vi "Data Chart for Flow Meter Test Time Chart.vi"(0 "Initialize":bool, 5 "Data Array":dbl[](array[numeric])) -> (6 "XY Graph":T1(graph))   [LabVIEW 2009]
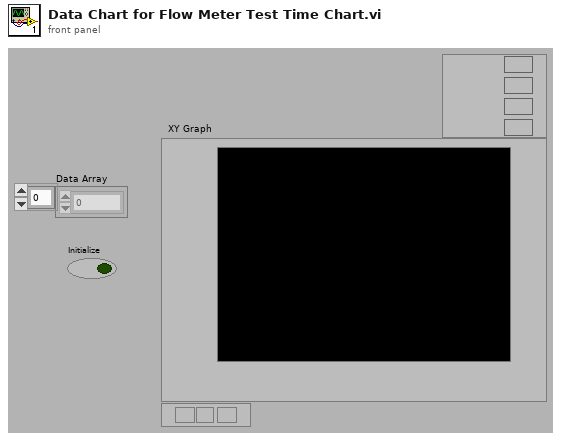
[diagram p1: front panel]
types:
  T1 = cluster{"XY chart data":cluster{"x":dbl, "y":dbl}[]}[]
  T2 = cluster{cluster{"Elapsed Time (sec)":dbl, dbl}[]}[]
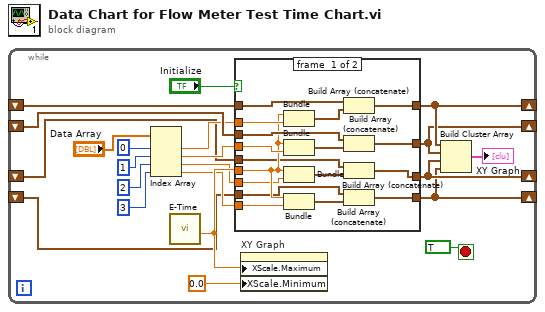
[diagram p0: block diagram]
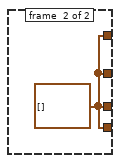
[diagram p2: hidden frame]
diagram:
  n1 = while {
    shift-right: [w21] -> _
    shift-left: _ -> [w19]
    shift-right: [w20] -> _
    shift-left: _ -> [w18]
    shift-right: [w3] -> _
    shift-left: _ -> [w5]
    shift-right: [w2] -> _
    shift-left: _ -> [w4]
    stop <- TRUE ("stop") stop-if-true
    n2 = Index Array(array="Data Array", index #1=0 ("index"), index #2=1 ("index"), index #3=2 ("index"), index #4=3 ("index")) -> (element #1=w10:dbl, element #2=w9:dbl, element #3=w7:dbl, element #4=w6:dbl)
    n3 = call "E-Time.vi"() -> ("Elapsed Time (sec)"=w8:dbl)  [unwired: 9 in, 2 out]
    n4 = case shown="False" "Initialize" {
      tunnel: [w37 w40] -> w21
      tunnel: [w36 w40] -> w20
      tunnel: w19 -> [w35 _]
      tunnel: w18 -> [w34 _]
      tunnel: w10 -> [w33 _]
      tunnel: w9 -> [w32 _]
      tunnel: w8 -> [w31 _]
      tunnel: w7 -> [w30 _]
      tunnel: w6 -> [w29 _]
      tunnel: w5 -> [w28 _]
      tunnel: w4 -> [w25 _]
      tunnel: [w24 w40] -> w3
      tunnel: [w23 w40] -> w2
      frame #0 {
        n5 = Bundle("Elapsed Time (sec)"=w31, w33) -> (w39:cluster{"Elapsed Time (sec)":dbl, dbl})  [unwired: 1 in]
        n6 = Bundle("Elapsed Time (sec)"=w31, w32) -> (w38:cluster{"Elapsed Time (sec)":dbl, dbl})  [unwired: 1 in]
        n7 = Bundle("Elapsed Time (sec)"=w31, w30) -> (w27:cluster{"Elapsed Time (sec)":dbl, dbl})  [unwired: 1 in]
        n8 = Bundle("Elapsed Time (sec)"=w31, w29) -> (w26:cluster{"Elapsed Time (sec)":dbl, dbl})  [unwired: 1 in]
        n9 = Build Array (concatenate)(w35, w39) -> (w37:cluster{"Elapsed Time (sec)":dbl, dbl}[])
        n10 = Build Array (concatenate)(w34, w38) -> (w36:cluster{"Elapsed Time (sec)":dbl, dbl}[])
        n11 = Build Array (concatenate)(w28, w27) -> (w24:cluster{"Elapsed Time (sec)":dbl, dbl}[])
        n12 = Build Array (concatenate)(w25, w26) -> (w23:cluster{"Elapsed Time (sec)":dbl, dbl}[])
      }
      frame #1 {
        w40 = cluster{"Elapsed Time (sec)":dbl, dbl}[] []
      }
    }
    n13 = property on="XY Graph" class="XYGraph (strict)"("XScale.Maximum"=w8, "XScale.Minimum"=0.0 ("X Scale.Range:Minimum")) -> ()  [unwired: 2 in, 2 out]
    n14 = Build Cluster Array(w21, w20, w3, w2) -> (→"XY Graph":T2)
  }
